vi "Load Workspace.vi"(8 "error in (no error)":errorcluster, 11 "Cfg Grandmaster in":refnum<class "Cfg Grandmaster.lvclass">) -> (0 "error out":errorcluster, 3 "Cfg Grandmaster out":refnum<class "Cfg Grandmaster.lvclass">)   [LabVIEW 2012, in "Configuration Grandmaster.lvlib" / "Cfg Grandmaster.lvclass"]
uses:
  Cfg Grandmaster.lvclass
  Common/Controls/Workspace.ctl
  Common/Controls/TCP Ports.ctl
  Common/Controls/Chassis Cfg Assoc.ctl
  Cfg Grandmaster.lvclass/Cfg Grandmaster.ctl
  Class Chassis BOM/Chassis BOM.lvclass/Chassis BOM.ctl
  TCP Server/TCP Connection Messages/Update Port Msg/Update Port Msg.lvclass/Update Port Msg.ctl
  <vilib>/ActorFramework/Message Enqueuer/Message Enqueuer.lvclass/Message Enqueuer.ctl
  Class Chassis BOM/Read Chassis Alias.vi
  <vilib>/ActorFramework/Message Enqueuer/Enqueue.vi
  <userlib>/GXML/_subVIis/GXML SearchParser/gxml_SearchParser.vi
  <vilib>/ActorFramework/Message Priority Queue/Priority Enqueue.vi
  TCP Server/TCP Connection Messages/Update Port Msg/Update Port Msg.lvclass
  Class Chassis BOM/Chassis BOM.lvclass
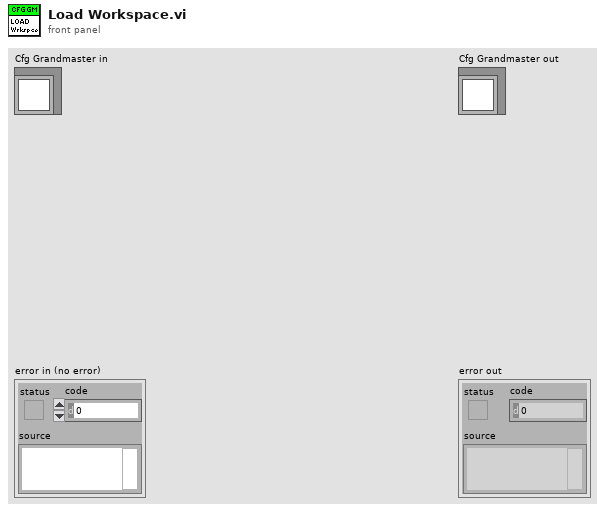
[diagram p1: front panel]
types:
  T1 = typedef "TCP Ports.ctl" = cluster{"Port Rdr":u16, "Port HS":u16, "Port LS":u16}
  T2 = typedef "Workspace.ctl" = cluster{"Ports":T1, "GlblConfig":T3[]}
  T3 = typedef "Chassis Cfg Assoc.ctl" = cluster{"Chassis Name":string, "CfgFile":path}
  T4 = typedef "ge_Cfg wChassis.ctl" = cluster{"Chassis BOM":refnum<class "Chassis BOM.lvclass">, "Chassis Cfg":refnum<class "ChassisCfg.lvclass">, "Chassis Tasks":refnum<class "Chassis Tasks.lvclass">, "HW Error":bool, "Unsvd Chgs?":bool}
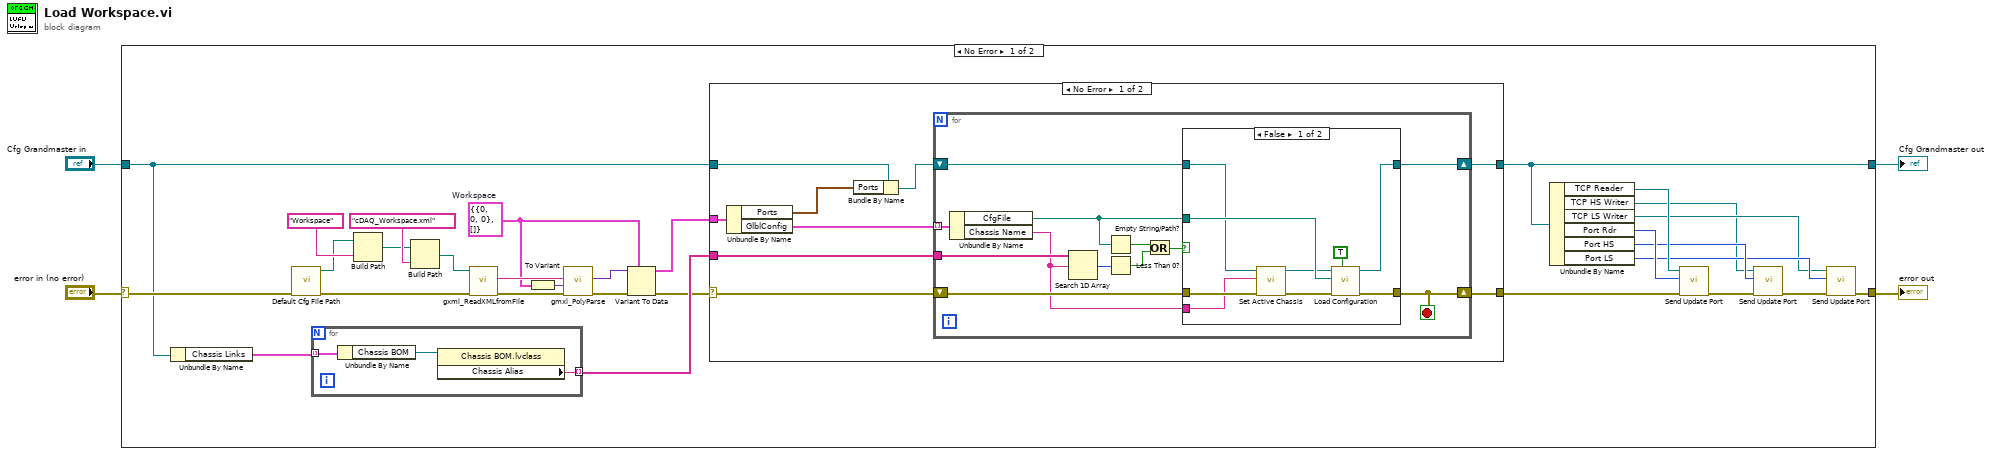
[diagram p0: block diagram]
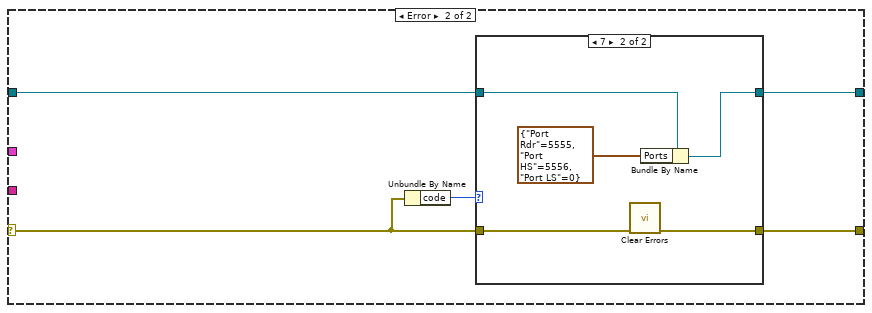
[diagram p3: hidden frame]
diagram:
  n1 = case shown="No Error" "error in (no error)" {
    selector: "error in (no error)" -> [w33 w82]
    tunnel: [w6 w82] -> w3
    tunnel: [w5 w81] -> w1
    tunnel: "Cfg Grandmaster in" -> [w16 w81]
    frame No Error {
      w19 = T2 {"Ports"={"Port Rdr"=0, "Port HS"=0, "Port LS"=0}, "GlblConfig"=[]}  # Workspace
      n2 = Unbundle By Name(w16) -> ("Chassis Links"=w32:T4[])
      n3 = call "Default Cfg File Path.vi"("error in (no error)"=w33) -> ("error out"=w17:errorcluster, "Default Path"=w23:path)  [unwired: 9 in]
      n4 = for {
        tunnel: w32 -> [w80] mode=indexing
        tunnel: [w78] -> w26 mode=indexing
        n5 = Unbundle By Name(w80) -> ("Chassis BOM"=w79:refnum<class "Chassis BOM.lvclass">)
        n6 = property class="Chassis BOM.lvclass"(reference=w79) -> ("Chassis Alias"=w78:string)  [unwired: 1 in, 2 out]
      }
      n7 = Build Path(base path=w23, name or relative path="Workspace") -> (appended path=w21:path)
      n8 = Build Path(base path=w21, name or relative path="cDAQ_Workspace.xml") -> (appended path=w20:path)
      n9 = call <userlib>:"gxml_ReadXMLfromFile.vi"("error in"=w17, "XML File Path"=w20) -> ("error out"=w27:errorcluster, "XML String Out"=w28:string)  [unwired: 7 in, 1 out]
      n10 = To Variant(anything=w19) -> (Variant=w29:variant)
      n11 = call-poly <userlib>:"gmxl_PolyParse.vi"("error in"=w27, "TypeDesc"=w29, "XML String In"=w28) -> ("error out"=w30:errorcluster, "Parsed Data"=w31:variant)  [unwired: 7 in]
      n12 = Variant To Data(error in=w30, type=w19, Variant=w31) -> (data=w18:T2, error out=w25:errorcluster)
      n13 = case shown="No Error" w25 {
        selector: w25 -> [w41 w69]
        tunnel: [w38 w70] -> w7
        tunnel: w26 -> [w42 _]
        tunnel: w18 -> [w40 _]
        tunnel: w16 -> [w36 w67]
        tunnel: [w37 w66] -> w5
        frame No Error {
          n14 = Unbundle By Name(w40) -> ("Ports"=w35:T1, "GlblConfig"=w39:T3[])
          n15 = Bundle By Name(cluster=w36, "Ports"=w35) -> (w34:refnum<class "Cfg Grandmaster.lvclass">)
          n16 = for {
            tunnel: w39 -> [w54] mode=indexing
            tunnel: w42 -> [w50]
            shift-right: [w52] -> w38
            shift-left: w41 -> [w53]
            shift-right: [w43] -> w37
            shift-left: w34 -> [w44]
            stop <- w52 stop-if-true
            n17 = Unbundle By Name(w54) -> ("CfgFile"=w51:path, "Chassis Name"=w49:string)
            n18 = Search 1D Array(1D array=w50, element=w49) -> (index of element=w48:i32)  [unwired: 1 in]
            n19 = Empty String/Path?(string/path=w51) -> (empty?=w47:bool)
            n20 = Less Than 0?(x=w48) -> (x < 0?=w46:bool)
            n21 = Or(x=w47, y=w46) -> (x .or. y?=w45:bool)
            n22 = case shown="False" w45 {
              tunnel: w53 -> [w63 w65]
              tunnel: [w60 w65] -> w52
              tunnel: w49 -> [w62 _]
              tunnel: w51 -> [w59 _]
              tunnel: w44 -> [w57 w64]
              tunnel: [w56 w64] -> w43
              frame False {
                n23 = call "Set Active Chassis.vi"("error in (no error)"=w63, "Chassis Name"=w62, "Cfg Grandmaster in"=w57) -> ("error out"=w61:errorcluster, "Cfg Grandmaster out"=w58:refnum<class "Cfg Grandmaster.lvclass">)  [unwired: 7 in]
                n24 = call "Load Configuration.vi"("Cursor Already Busy?"=TRUE, "error in (no error)"=w61, "Config File to Load"=w59, "Cfg Grandmaster in"=w58) -> ("error out"=w60:errorcluster, "Cfg Grandmaster out"=w56:refnum<class "Cfg Grandmaster.lvclass">)  [unwired: 6 in]
              }
              frame True {
              }
            }
          }
        }
        frame Error {
          n25 = Unbundle By Name(w69) -> ("code"=w68:i32)
          n26 = case shown="7" w68 {
            tunnel: w69 -> [w72 w77]
            tunnel: [w72 w76] -> w70
            tunnel: w67 -> [w71 w75]
            tunnel: [w71 w73] -> w66
            frame Default {
            }
            frame 7 {
              n27 = call <vilib>:"Clear Errors.vi"("error in (no error)"=w77) -> ("error out"=w76:errorcluster)  [unwired: 6 in]
              n28 = Bundle By Name(cluster=w75, "Ports"=T1 {"Port Rdr"=5555, "Port HS"=5556, "Port LS"=0}) -> (w73:refnum<class "Cfg Grandmaster.lvclass">)
            }
          }
        }
      }
      n29 = Unbundle By Name(w5) -> ("TCP Reader"=w14:refnum<class "Message Enqueuer.lvclass">, "TCP HS Writer"=w9:refnum<class "Message Enqueuer.lvclass">, "TCP LS Writer"=w10:refnum<class "Message Enqueuer.lvclass">, "Port Rdr"=w15:u16, "Port HS"=w12:u16, "Port LS"=w11:u16)
      n30 = call "Send Update Port.vi"("error in (no error)"=w7, "Port"=w15, "Message Enqueuer"=w14) -> ("error out"=w13:errorcluster)  [unwired: 7 in, 1 out]
      n31 = call "Send Update Port.vi"("error in (no error)"=w13, "Port"=w12, "Message Enqueuer"=w9) -> ("error out"=w8:errorcluster)  [unwired: 7 in, 1 out]
      n32 = call "Send Update Port.vi"("error in (no error)"=w8, "Port"=w11, "Message Enqueuer"=w10) -> ("error out"=w6:errorcluster)  [unwired: 7 in, 1 out]
    }
    frame Error {
    }
  }
  "error out" <- w3
  "Cfg Grandmaster out" <- w1
